vi "findZref.vi"(10 "aTarget":cluster{"Xvalues":dbl[], "Yvalues":dbl[]}={"Xvalues"=[1.040926042556437, 1.0312252179740482, 1.0211896176877788, 1.0107916504073806, 1.0, 0.9887789066622864, 0.9770872631810879, 0.9648774654735645, 0.9520939317160783, 0.9386711670518244, 0.9245311936078002, 0.9095800754352008, 0.8937031220268912, 0.8767581097958107, 0.8585654364377537, 0.8388933525508411, 0.8174349420135516, 0.7937705277401984, 0.7673026110088009, 0.7371346086455506], "Yvalues"=[600.0, 575.0, 550.0, 525.0, 500.0, 475.0, 450.0, 425.0, 400.0, 375.0, 350.0, 325.0, 300.0, 275.0, 250.0, 225.0, 200.0, 175.0, 150.0, 125.0]}) -> (1 "Zref":dbl)   [LabVIEW 2018]
panel:
  out "fractional index or x":dbl
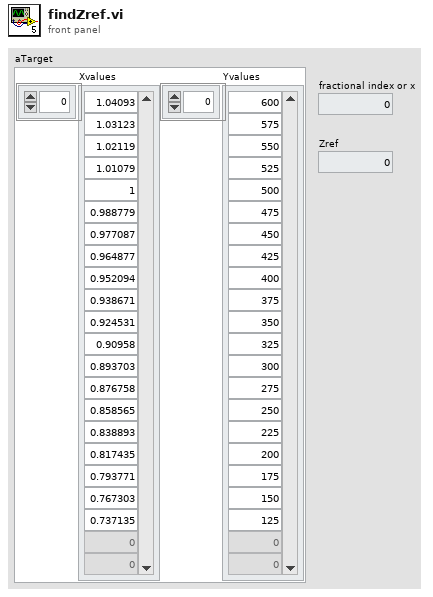
[diagram p1: front panel]
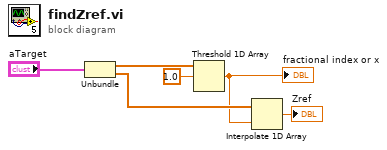
[diagram p0: block diagram]
diagram:
  n1 = Unbundle("aTarget") -> ("Xvalues"=w5:dbl[], "Yvalues"=w3:dbl[])
  n2 = Threshold 1D Array(2:1.0 ("fractional index or x"), 3:w5) -> (0:w2:dbl)  [unwired: 1 in]
  "fractional index or x" <- w2
  n3 = Interpolate 1D Array(1:w2, 2:w3) -> (0:→"Zref":dbl)
